vi "StringToIntArray.vi"(3 "InputString":string) -> (0 "AllNumbers?":bool, 1 "OutArray":i32[](array[numeric]))   [LabVIEW 2022 SP3]
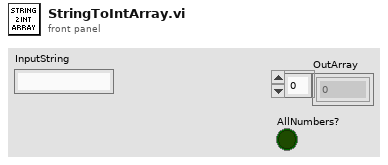
[diagram p1: front panel]
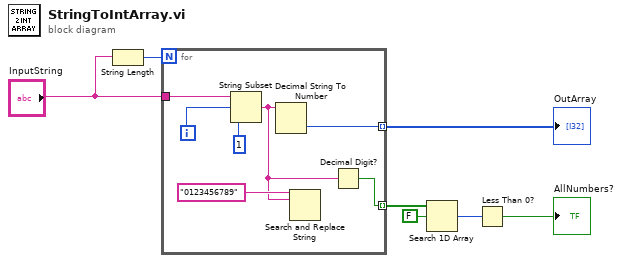
[diagram p0: block diagram]
diagram:
  n1 = String Length(string="InputString") -> (length=w7:i32)
  n2 = for {
    N: w7 -> [_]
    tunnel: "InputString" -> [w14]
    tunnel: [w11] -> w5 mode=indexing
    tunnel: [w8] -> w4 mode=indexing
    i -> [w13]
    n3 = String Subset(string=w14, offset (0)=w13, length (rest)=1 ("length (rest)")) -> (substring=w9:string)
    n4 = Decimal String To Number(string=w9) -> (number=w11:i32)  [unwired: 2 in, 1 out]
    n5 = Search and Replace String(input string="0123456789", search string=w9) -> ()  [unwired: 6 in, 4 out]
    n6 = Decimal Digit?(1:w9) -> (0:w8:bool)
  }
  "OutArray" <- w5
  n7 = Search 1D Array(1D array=w4, element=FALSE) -> (index of element=w2:i32)  [unwired: 1 in]
  n8 = Less Than 0?(x=w2) -> (x < 0?=→"AllNumbers?":bool)
